vi "Write Active measurements enqueuers.vi"(8 "error in (no error)":errorcluster, 10 "Active measurements enqueuers":refnum<class "Message Enqueuer.lvclass">[](array[class]), 11 "Measure Controller in":refnum<class "Measure Controller.lvclass">) -> (0 "error out":errorcluster, 3 "Measure Controller out":refnum<class "Measure Controller.lvclass">)   [LabVIEW 2015, in "Measure Controller.lvclass"]
uses:
  Measure Controller.lvclass
  <vilib>/ActorFramework/Message Enqueuer/Message Enqueuer.lvclass
  Measure Controller.lvclass/Measure Controller.ctl
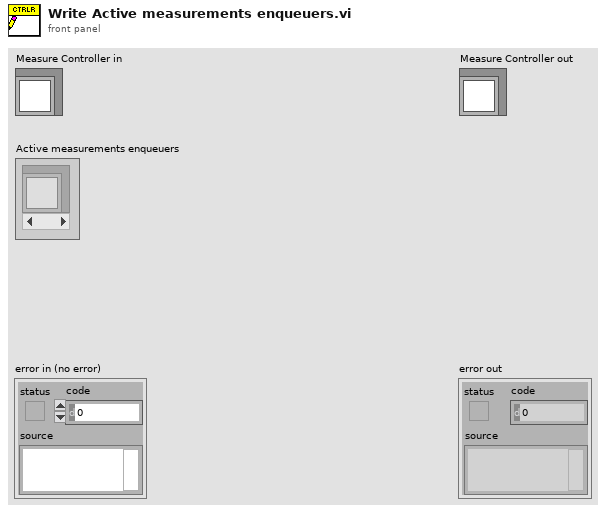
[diagram p1: front panel]
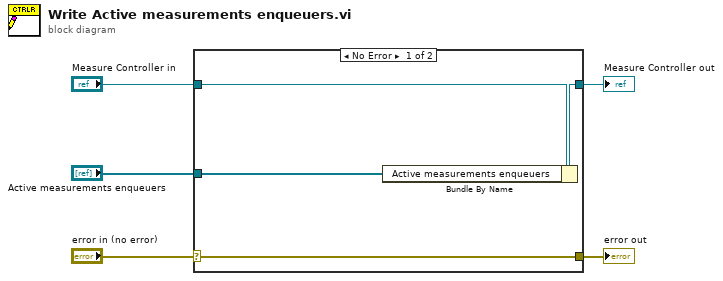
[diagram p0: block diagram]
diagram:
  n1 = case shown="No Error" "error in (no error)" {
    selector: "error in (no error)" -> [w9 w10]
    tunnel: [w9 w10] -> w4
    tunnel: [w7 w11] -> w2
    tunnel: "Measure Controller in" -> [w8 w11]
    tunnel: "Active measurements enqueuers" -> [w6 _]
    frame No Error {
      n2 = Bundle By Name(cluster=w8, "Active measurements enqueuers"=w6) -> (w7:refnum<class "Measure Controller.lvclass">)
    }
    frame Error {
    }
  }
  "error out" <- w4
  "Measure Controller out" <- w2
